vi "resizeControl.vi"(8 "error in (no error)":errorcluster, 11 "Topic in":refnum<class "Topic.lvclass">) -> (0 "error out":errorcluster, 3 "Topic out":refnum<class "Topic.lvclass">)   [LabVIEW 2013, in "Topic.lvclass"]
uses:
  Topic.lvclass
  Topic.lvclass/Topic.ctl
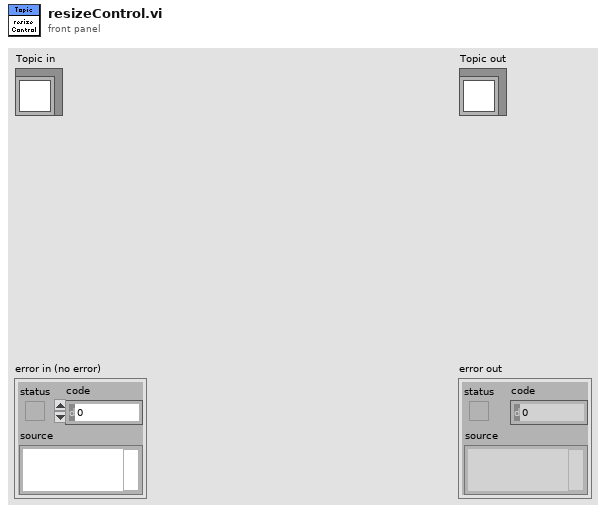
[diagram p1: front panel]
types:
  T1 = typedef "LVRectTypeDef.ctl" = cluster{"Left":i16, "Top":i16, "Right":i16, "Bottom":i16}
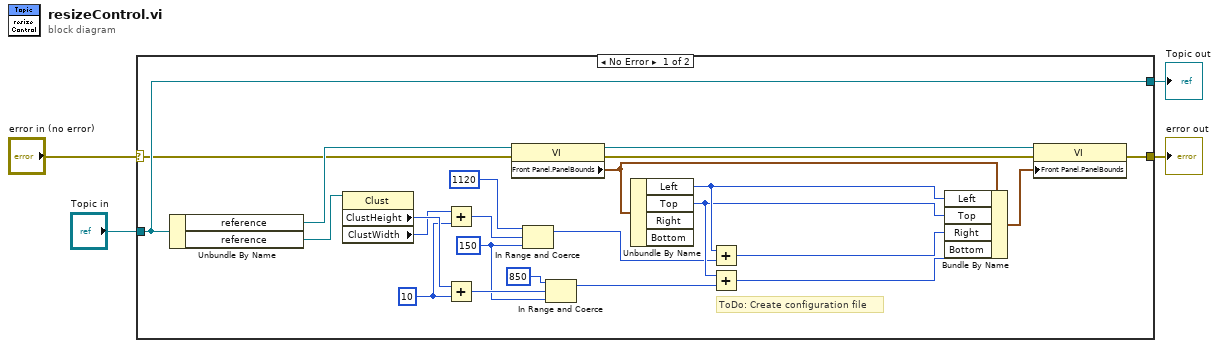
[diagram p0: block diagram]
diagram:
  n1 = case shown="No Error" "error in (no error)" {
    selector: "error in (no error)" -> [w13 w29]
    tunnel: [w12 w29] -> w3
    tunnel: [w14 w28] -> w1
    tunnel: "Topic in" -> [w14 w28]
    frame No Error {
      w7 = u32 150 ("lower limit")
      w21 = u32 10 ("y")
      # "ToDo: Create configuration file"
      n2 = Unbundle By Name(w14) -> ("reference"=w17:refnum<vi>, "reference"=w27:refnum<vi>)
      n3 = property class="Clust"(reference=w27) -> ("ClustHeight"=w22:u32, "ClustWidth"=w19:u32)  [unwired: 1 in, 2 out]
      n4 = Add(x=w19, y=w21) -> (x+y=w11:u32)
      n5 = Add(x=w22, y=w21) -> (x+y=w9:u32)
      n6 = property class="VI"(reference=w17, error in=w13) -> (reference out=w26:refnum<vi>, error out=w25:errorcluster, "Front Panel.PanelBounds"=w24:T1)
      n7 = In Range and Coerce(upper limit=u32 1120, x=w11, lower limit=w7) -> (coerced(x)=w6:u32)  [unwired: 1 out]
      n8 = In Range and Coerce(upper limit=u32 850, x=w9, lower limit=w7) -> (coerced(x)=w5:u32)  [unwired: 1 out]
      n9 = Unbundle By Name(w24) -> ("Left"=w16:i16, "Top"=w15:i16)  [unwired: 2 out]
      n10 = Add(x=w16, y=w6) -> (x+y=w18:u32)
      n11 = Add(x=w15, y=w5) -> (x+y=w20:u32)
      n12 = Bundle By Name(cluster=w24, "Left"=w16, "Top"=w15, "Right"=w18, "Bottom"=w20) -> (w23:T1)
      n13 = property class="VI"(reference=w26, error in=w25, "Front Panel.PanelBounds"=w23) -> (error out=w12:errorcluster)  [unwired: 1 out]
    }
    frame Error {
    }
  }
  "error out" <- w3
  "Topic out" <- w1
